vi "EXP 1.vi"() -> ()   [LabVIEW 2018]
panel:
  out "power consumed\n       WATTS":dbl
  out "OVERALL TIIME M.SECS":i32
  out "Alert C2":string
  out "Alert L1":string
  out "Alert L2":string
  out "alertc1":string
  out "Alaramc2":bool
  out "alaraml1":bool
  out "Alaraml2":bool
  out "Alaramc1":bool
  in  "stop 2":bool
  out "LIGHT1 5 POWER":dbl
  out "LIGHT1 4 POWER":dbl
  out "LIGHT23 POWER":dbl
  out "LIGHT1 2 POWER":dbl
  out "OVERALL ENERGY\nCONSUMED":dbl
  out "LAB-1 OVERALL POWER":dbl
  out "LAB-1 OVERALL TIME":i32
  out "LAB-2 OVERALL POWER":dbl
  out "LAB-2 OVERALL TIME":i32
  out "LIGHT 12 TIME":i32 format="%<%H:%M>t"
  out "LIGHT23 TIME":i32 format="%<%H:%M>t"
  out "LIGHT1 4 TIME":i32 format="%<%H:%M>t"
  out "LIGHT1 5 TIME":i32 format="%<%H:%M>t"
  out "FAN13 POWER":dbl
  out "FAN3 POWER":dbl
  out "FAN15 POWER":dbl
  out "FAN5 POWER":dbl
  out "FAN5 TIME":i32
  out "FAN1 5 TIME":i32
  out "FAN3 TIME":i32
  out "FAN13 TIME":i32
  out "FAN1 4":dbl
  out "FAN4":dbl
  out "LIGHT23 2":dbl
  out "LIGHT1 3":dbl
  out "FAN1 4 TIME":i32
  out "FAN4 TIME":i32
  out "LIGHT23 2 TIME":i32
  out "LIGHT 1 3 TIME":i32
  out "CLASS-2 OVERALL TIIME":i32
  out "CLASS-2 POWER OUTPUT":dbl
  out "DAY":string
  out "lighht1 5":bool
  out "lighht1 4":bool
  out "fan 5":bool
  out "fan1 5":bool
  out "light23 2":bool
  out "lighht1 3":bool
  out "fan 4":bool
  out "fan1 4":bool
  out "light23":bool
  out "lighht1 2":bool
  out "fan 3":bool
  out "fan1 3":bool
  out "current time":timestamp
  out "INDICATED VALUE":dbl
  out "light 2 time\nHH:MM 2":i32 caption="light 2 time" format="%<%H:%M>t"
  out "light 1 time\nHH:MM  2":i32 caption="light 2 time" format="%<%H:%M>t"
  out "fan 1 time\nHH:MM   2":i32 caption="light 2 time" format="%<%H:%M>t"
  out "fan 2 time\nHH:MM  2":i32 caption="light 2 time" format="%<%H:%M>t"
  out "light 2 output 2":dbl
  out "light 1 output  2":dbl
  out "fan 1 output  2":dbl
  out "fan 2 output  2":dbl
  out "Alert Overall":string
  out "CLASS 1 OVERALL TIME\nHH:MM  2":i32 caption="light 2 time" format="%<%H:%M>t"
  out "CLASS-1 POWER OUTPUT":dbl
  out "ALARM INDICATOR":bool
  out "light2 2":bool
  out "lighht1":bool
  out "fan 2":bool
  out "fan1 2":bool
  # "PRE"
  # "LAB-1"
  # "CLASS-1 DATA"
  # "CLASS 2"
  # "CLASS1"
  # "LAB-2"
  # "###############################################################"
  # "LAB-1 DATA"
  # "###############################################################"
  # "LAB-2"
  # "#\n#\n#\n#\n#\n#\n#\n#\n#\n#\n#\n#\n#\n#\n#\n#\n#\n#\n#\n#\n#\n#\n#\n#\n#\n#\n#\n#\n#\n#"
  # "##TIME AND POWER OF INDIVIDUAL CLASS ROOMS AND LABS##"
  # "###############################################################"
  # "CLASS-2"
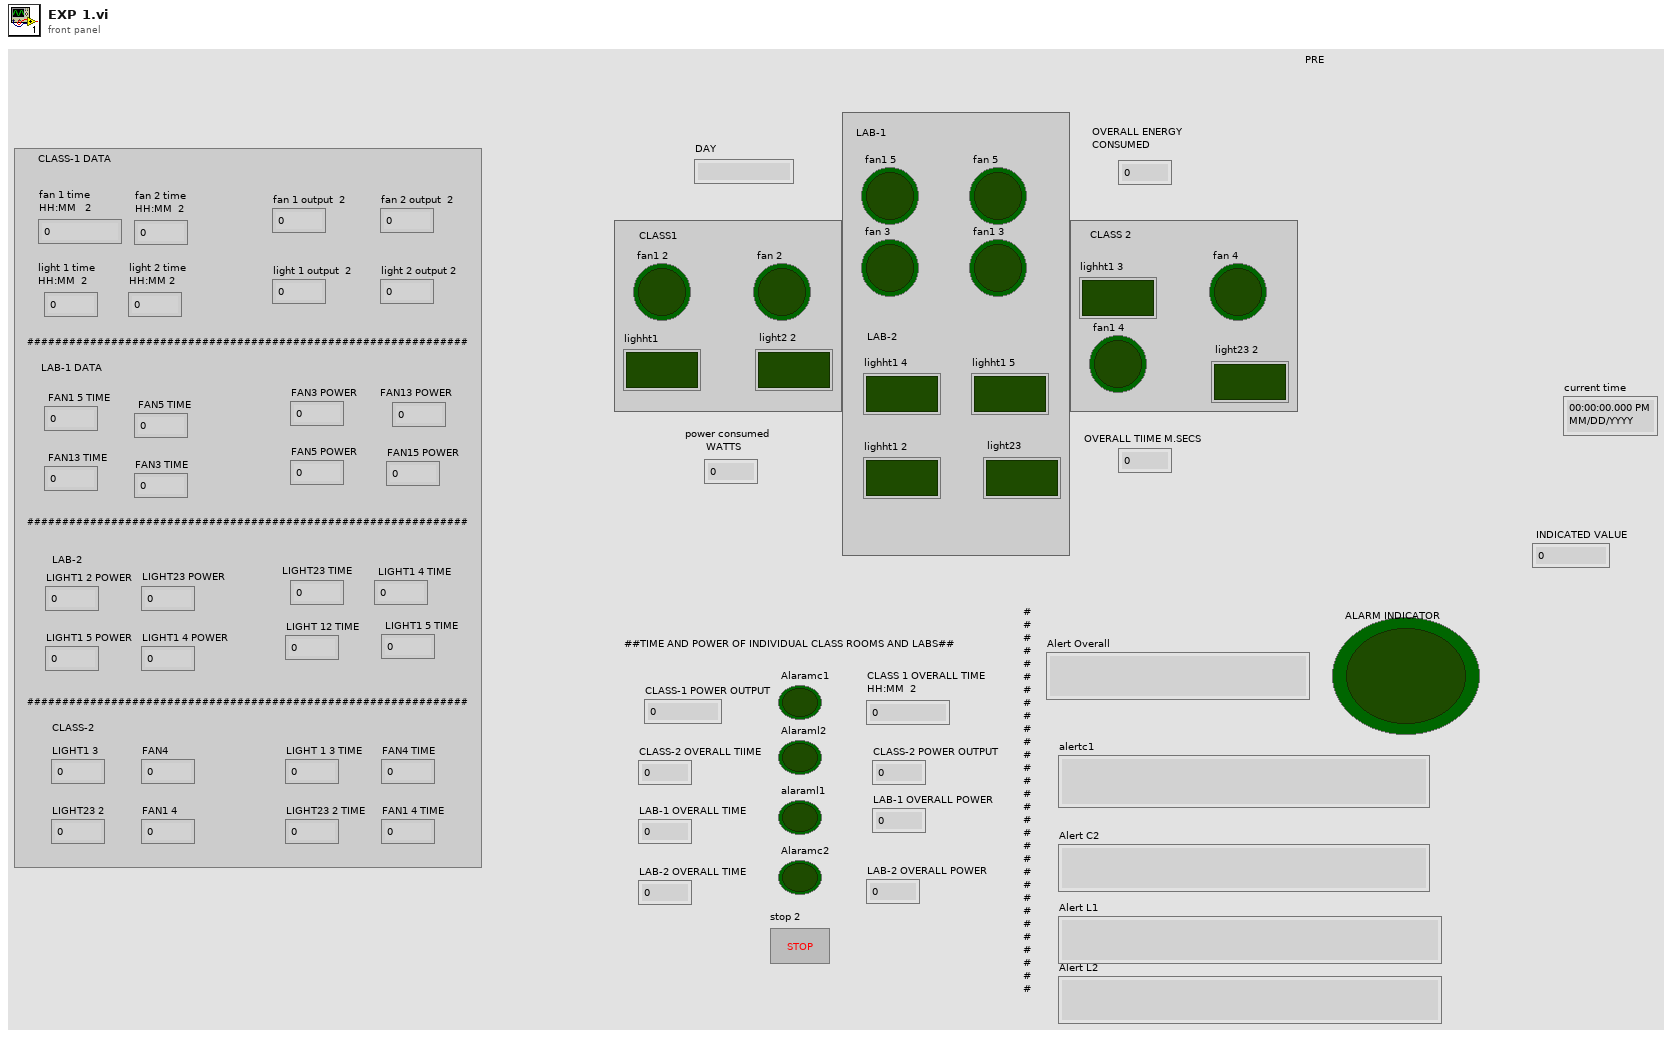
[diagram p1: front panel]
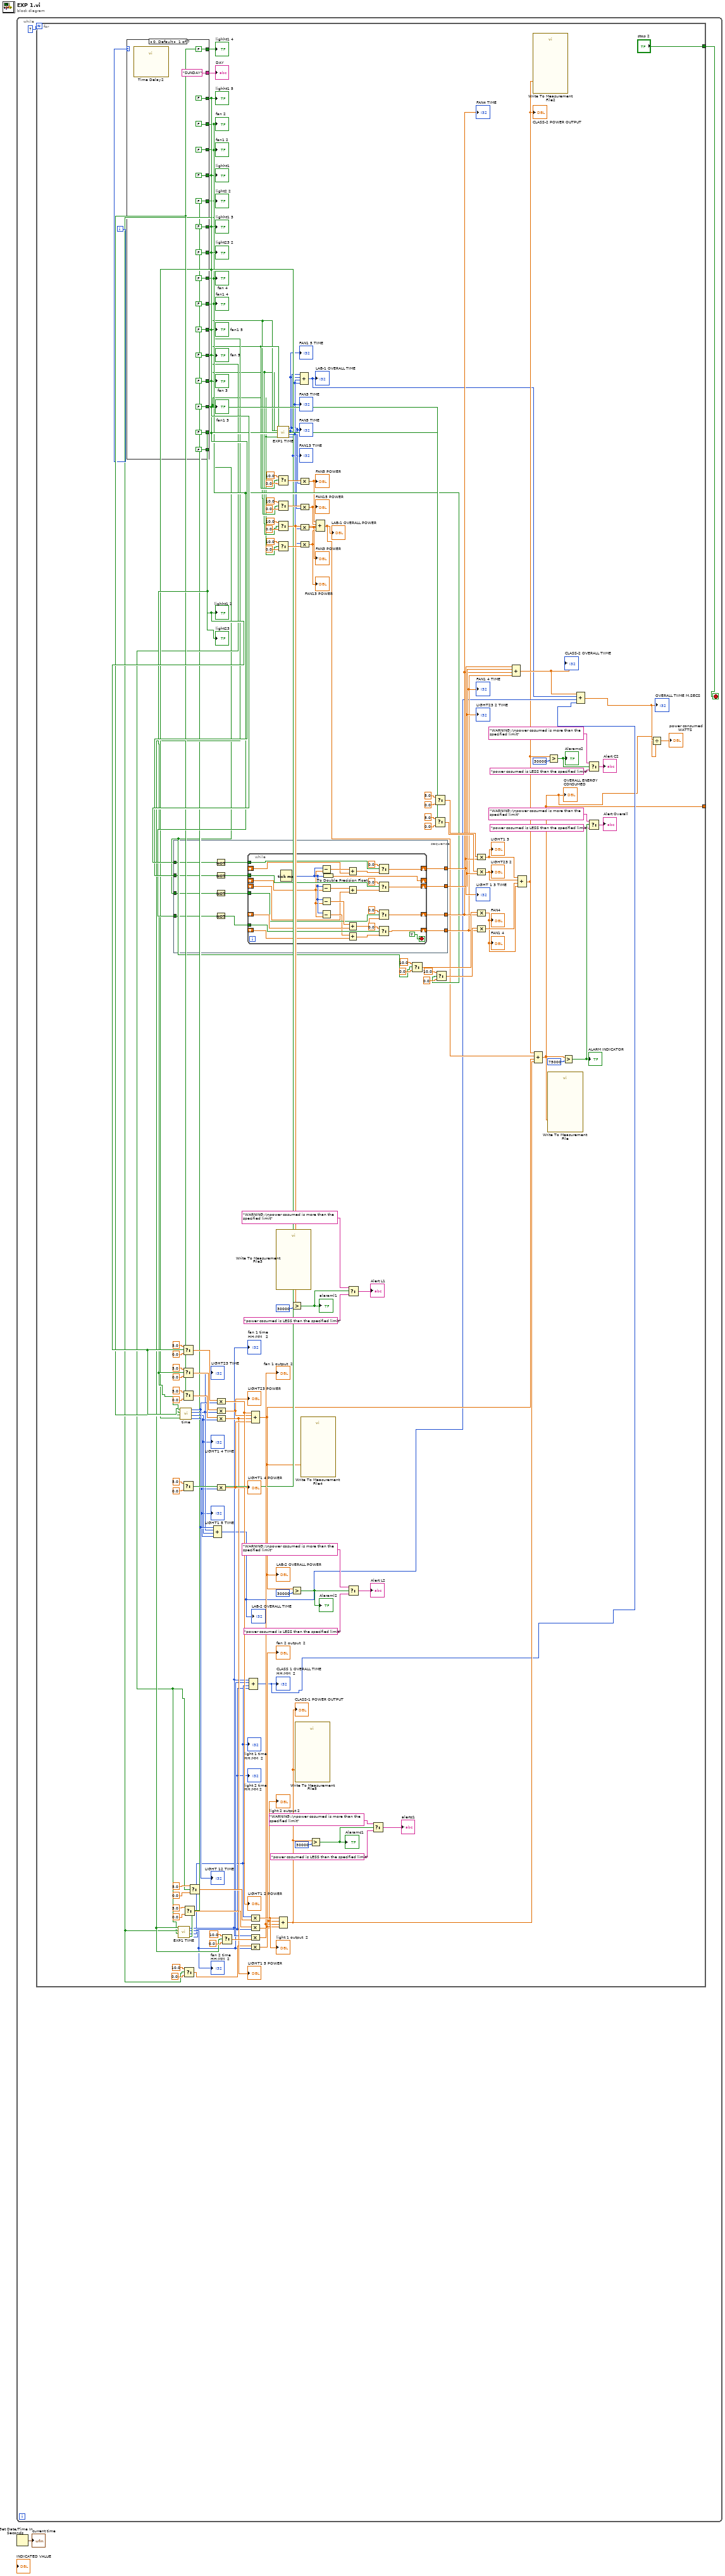
[diagram p0: block diagram]
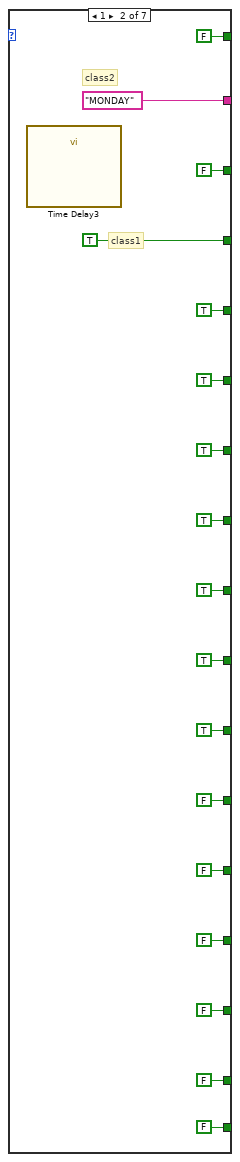
[diagram p2: hidden frame]
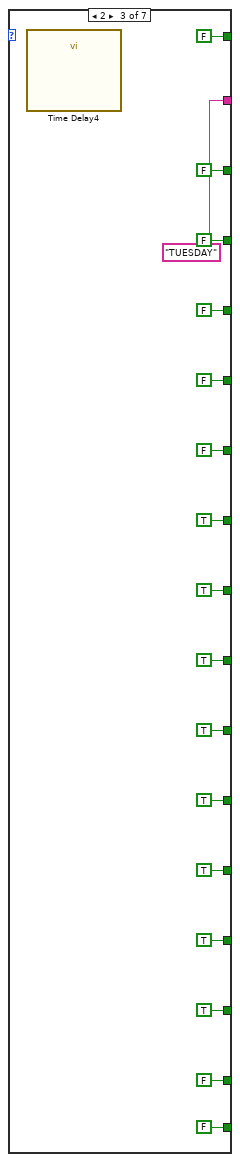
[diagram p3: hidden frame]
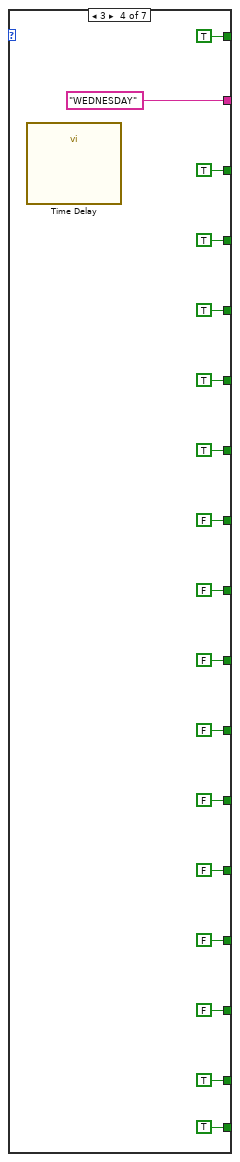
[diagram p4: hidden frame]
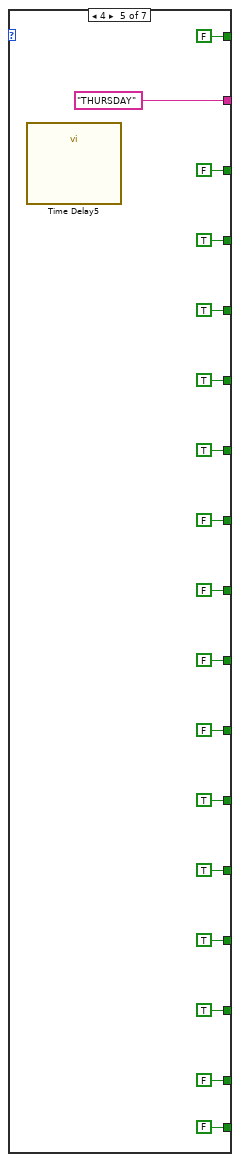
[diagram p5: hidden frame]
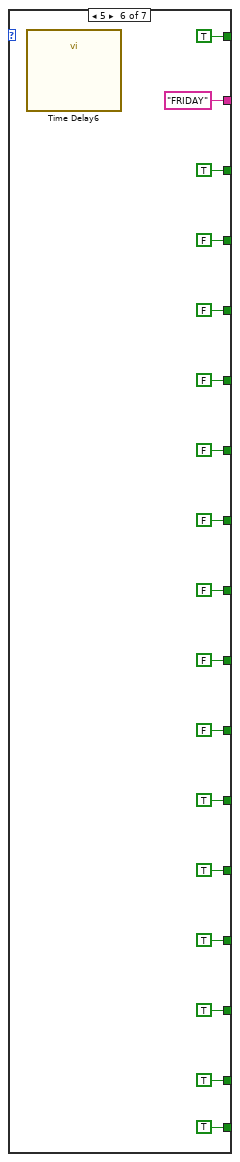
[diagram p6: hidden frame]
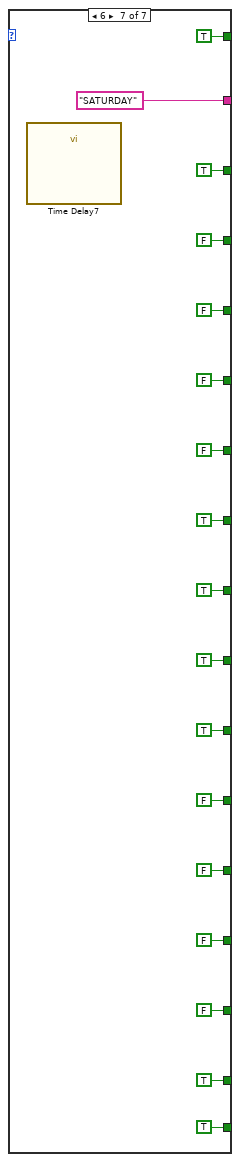
[diagram p7: hidden frame]
diagram:
  n1 = while {
    stop <- w2 stop-if-true
    n2 = for {
      N: 7 -> [_]
      tunnel: [w16] -> _
      tunnel: ["stop 2"] -> w2
      i -> [w54]
      n3 = case shown="0, Default" w54 {
        tunnel: [FALSE ("Boolean 9") TRUE ("Boolean 9") FALSE ("Boolean 9") TRUE ("Boolean 9") TRUE ("Boolean 8") FALSE ("Boolean 8") FALSE ("Boolean 8")] -> w53
        tunnel: [FALSE ("Boolean 11") TRUE ("Boolean 8") FALSE ("Boolean 11") TRUE ("Boolean 11") TRUE ("Boolean 8") FALSE ("Boolean 8") FALSE ("Boolean 8")] -> w52
        tunnel: [FALSE ("Boolean 8") TRUE ("Boolean 11") FALSE ("Boolean 8") TRUE ("Boolean 8") TRUE ("Boolean 8") FALSE ("Boolean 8") FALSE ("Boolean 8")] -> w51
        tunnel: [FALSE ("Boolean 10") TRUE ("Boolean 10") FALSE ("Boolean 10") TRUE ("Boolean 10") TRUE ("Boolean 8") FALSE ("Boolean 8") FALSE ("Boolean 8")] -> w50
        tunnel: [FALSE ("Boolean 8") TRUE ("Boolean 9") TRUE ("Boolean 9") FALSE ("Boolean 8") FALSE ("Boolean 8") FALSE ("Boolean 8") TRUE ("Boolean 8")] -> w110
        tunnel: [FALSE ("Boolean 8") TRUE ("Boolean 9") TRUE ("Boolean 9") FALSE ("Boolean 8") FALSE ("Boolean 8") FALSE ("Boolean 8") TRUE ("Boolean 8")] -> w109
        tunnel: [FALSE ("Boolean 8") TRUE ("Boolean 8") TRUE ("Boolean 8") FALSE ("Boolean 8") FALSE ("Boolean 8") FALSE ("Boolean 8") TRUE ("Boolean 8")] -> w6
        tunnel: [FALSE ("Boolean 8") TRUE ("Boolean 8") TRUE ("Boolean 8") FALSE ("Boolean 8") FALSE ("Boolean 8") FALSE ("Boolean 8") TRUE ("Boolean 8")] -> w88
        tunnel: [FALSE ("Boolean 9") FALSE ("Boolean 9") TRUE ("Boolean 9") FALSE ("Boolean 9") TRUE ("Boolean 8") TRUE ("Boolean 8") FALSE ("Boolean 8")] -> w13
        tunnel: [FALSE ("Boolean 9") FALSE ("Boolean 9") TRUE ("Boolean 9") FALSE ("Boolean 9") TRUE ("Boolean 8") TRUE ("Boolean 8") FALSE ("Boolean 8")] -> w14
        tunnel: [FALSE ("Boolean 9") FALSE ("Boolean 9") TRUE ("Boolean 9") FALSE ("Boolean 9") TRUE ("Boolean 8") TRUE ("Boolean 8") FALSE ("Boolean 8")] -> w12
        tunnel: [FALSE ("Boolean 9") FALSE ("Boolean 9") TRUE ("Boolean 9") FALSE ("Boolean 9") TRUE ("Boolean 8") TRUE ("Boolean 8") FALSE ("Boolean 8")] -> w11
        tunnel: [FALSE ("Boolean 8") FALSE ("Boolean 8") FALSE ("Boolean 8") TRUE ("Boolean 8") FALSE ("Boolean 8") TRUE ("Boolean 8") TRUE ("Boolean 8")] -> w75
        tunnel: [FALSE ("Boolean 8") FALSE ("Boolean 8") FALSE ("Boolean 8") TRUE ("Boolean 8") FALSE ("Boolean 8") TRUE ("Boolean 8") TRUE ("Boolean 8")] -> w74
        tunnel: [FALSE ("Boolean 8") FALSE ("Boolean 8") FALSE ("Boolean 8") TRUE ("Boolean 8") FALSE ("Boolean 8") TRUE ("Boolean 8") TRUE ("Boolean 8")] -> w73
        tunnel: [FALSE ("Boolean 8") FALSE ("Boolean 8") FALSE ("Boolean 8") TRUE ("Boolean 8") FALSE ("Boolean 8") TRUE ("Boolean 8") TRUE ("Boolean 8")] -> w72
        tunnel: ["SUNDAY" "MONDAY" "TUESDAY" "WEDNESDAY" "THURSDAY" "FRIDAY" "SATURDAY"] -> w119
        frame 0, Default {
          n4 = call "Time Delay2"() -> ()  [unwired: 11 in, 1 out]
        }
        frame 1 {
          # "class2"
          # "class1"
          n5 = call "Time Delay3"() -> ()  [unwired: 11 in, 1 out]
        }
        frame 2 {
          n6 = call "Time Delay4"() -> ()  [unwired: 11 in, 1 out]
        }
        frame 3 {
          n7 = call "Time Delay"() -> ()  [unwired: 11 in, 1 out]
        }
        frame 4 {
          n8 = call "Time Delay5"() -> ()  [unwired: 11 in, 1 out]
        }
        frame 5 {
          n9 = call "Time Delay6"() -> ()  [unwired: 11 in, 1 out]
        }
        frame 6 {
          n10 = call "Time Delay7"() -> ()  [unwired: 11 in, 1 out]
        }
      }
      "fan1 2" <- w53
      "fan 2" <- w52
      "lighht1" <- w51
      "light2 2" <- w50
      "fan1 3" <- w11
      "fan 3" <- w12
      "lighht1 2" <- w75
      "light23" <- w74
      "fan1 4" <- w88
      "fan 4" <- w6
      "lighht1 3" <- w110
      "light23 2" <- w109
      "fan1 5" <- w13
      "fan 5" <- w14
      "lighht1 4" <- w73
      "lighht1 5" <- w72
      "DAY" <- w119
      n11 = stacked-sequence {
        tunnel: [w148] -> w97
        tunnel: [w139] -> w98
        tunnel: [w150] -> w99
        tunnel: [w149] -> w100
        tunnel: w88 -> [w142]
        tunnel: w6 -> [w140]
        tunnel: w109 -> [w144]
        tunnel: w110 -> [w143]
        frame #0 {
          n12 = Not(x=w143) -> (.not. x?=w146:bool)
          n13 = Not(x=w144) -> (.not. x?=w147:bool)
          n14 = Not(x=w140) -> (.not. x?=w141:bool)
          n15 = Not(x=w142) -> (.not. x?=w145:bool)
          n16 = while {
            shift-right: [w165] -> w139
            shift-left: _ -> [w177]
            shift-right: [w175] -> _
            shift-left: _ -> [w151]
            tunnel: w141 -> [w173]
            tunnel: w145 -> [w169]
            tunnel: w146 -> [w168]
            tunnel: w147 -> [w167]
            shift-right: [w164] -> w148
            shift-left: _ -> [w158]
            shift-right: [w163] -> w149
            shift-left: _ -> [w156]
            shift-right: [w162] -> w150
            shift-left: _ -> [w154]
            stop <- TRUE stop-if-true
            n17 = Tick Count (ms)() -> (millisecond timer value=w152:u32)
            n18 = Subtract(x=w152, y=w151) -> (x-y=w161:dbl)
            n19 = Subtract(x=w152, y=w151) -> (x-y=w160:dbl)
            n20 = Subtract(x=w152, y=w151) -> (x-y=w178:dbl)
            n21 = Subtract(x=w152, y=w151) -> (x-y=w159:dbl)
            n22 = To Double Precision Float(number=w152) -> (double precision float=w175:dbl)
            n23 = Add(x=w161, y=w156) -> (x+y=w155:dbl)
            n24 = Add(x=w160, y=w154) -> (x+y=w153:dbl)
            n25 = Add(x=w178, y=w177) -> (x+y=w166:dbl)
            n26 = Add(x=w159, y=w158) -> (x+y=w157:dbl)
            n27 = Select(t=0.0, s=w168, f=w155) -> (s? t:f=w163:dbl)
            n28 = Select(t=0.0, s=w167, f=w153) -> (s? t:f=w162:dbl)
            n29 = Select(t=0.0, s=w173, f=w166) -> (s? t:f=w165:dbl)
            n30 = Select(t=0.0, s=w169, f=w157) -> (s? t:f=w164:dbl)
          }
        }
      }
      "LIGHT 1 3 TIME" <- w100
      "LIGHT23 2 TIME" <- w99
      "FAN4 TIME" <- w98
      "FAN1 4 TIME" <- w97
      n31 = call "EXP1 TIME.vi"("s 2"=w50, "s"=w51, "s 4"=w52, "s 3"=w53) -> ("time 2"=w46:i32, "time"=w47:i32, "time 4"=w48:i32, "time 3"=w49:i32)  [unwired: 4 in]
      "fan 1 time\nHH:MM   2" <- w49
      "fan 2 time\nHH:MM  2" <- w48
      "light 1 time\nHH:MM  2" <- w47
      "light 2 time\nHH:MM 2" <- w46
      n32 = call "time.vi"("s 2"=w72, "s"=w73, "s 4"=w74, "s 3"=w75) -> ("time 2"=w61:i32, "time"=w62:i32, "time 4"=w63:i32, "time 3"=w64:i32)  [unwired: 4 in]
      "LIGHT1 5 TIME" <- w61
      "LIGHT1 4 TIME" <- w62
      "LIGHT23 TIME" <- w63
      "LIGHT 12 TIME" <- w64
      n33 = Select(t=5.0, s=w75, f=0.0) -> (s? t:f=w71:dbl)
      n34 = Select(t=5.0, s=w74, f=0.0) -> (s? t:f=w70:dbl)
      n35 = Select(t=5.0, s=w73, f=0.0) -> (s? t:f=w69:dbl)
      n36 = Select(t=5.0, s=w72, f=0.0) -> (s? t:f=w68:dbl)
      n37 = Select(t=10.0, s=w52, f=0.0) -> (s? t:f=w55:dbl)
      n38 = Select(t=5.0, s=w50, f=0.0) -> (s? t:f=w56:dbl)
      n39 = Select(t=5.0, s=w51, f=0.0) -> (s? t:f=w136:dbl)
      n40 = Compound Arithmetic op=ADD(w64, w63, w62, w61) -> (w20:i32)
      "LAB-2 OVERALL TIME" <- w20
      n41 = Compound Arithmetic op=MULTIPLY(w71, w64) -> (w60:dbl)
      "LIGHT1 2 POWER" <- w60
      n42 = Compound Arithmetic op=MULTIPLY(w70, w63) -> (w59:dbl)
      "LIGHT23 POWER" <- w59
      n43 = Compound Arithmetic op=MULTIPLY(w69, w62) -> (w57:dbl)
      "LIGHT1 5 POWER" <- w57
      n44 = Compound Arithmetic op=MULTIPLY(w68, w61) -> (w58:dbl)
      "LIGHT1 4 POWER" <- w58
      n45 = Select(t=10.0, s=w53, f=0.0 ("t")) -> (s? t:f=w132:dbl)
      n46 = Compound Arithmetic op=ADD(w49, w48, w47, w46) -> (w19:i32)
      "CLASS 1 OVERALL TIME\nHH:MM  2" <- w19
      n47 = Compound Arithmetic op=ADD(w60, w59, w57, w58) -> (w23:dbl)
      "LAB-2 OVERALL POWER" <- w23
      n48 = Compound Arithmetic op=MULTIPLY(w47, w136) -> (w137:dbl)
      "light 1 output  2" <- w137
      n49 = Compound Arithmetic op=MULTIPLY(w56, w46) -> (w133:dbl)
      "light 2 output 2" <- w133
      n50 = Compound Arithmetic op=MULTIPLY(w49, w132) -> (w134:dbl)
      "fan 1 output  2" <- w134
      n51 = Compound Arithmetic op=MULTIPLY(w55, w48) -> (w135:dbl)
      "fan 2 output  2" <- w135
      n52 = call "EXP1 TIME.vi"("s 2"=w11, "s"=w12, "s 4"=w13, "s 3"=w14) -> ("time 2"=w8:i32, "time"=w9:i32, "time 4"=w5:i32, "time 3"=w10:i32)  [unwired: 4 in]
      "FAN13 TIME" <- w8
      "FAN3 TIME" <- w9
      "FAN1 5 TIME" <- w5
      "FAN5 TIME" <- w10
      n53 = Select(t=10.0, s=w14, f=0.0) -> (s? t:f=w79:dbl)
      n54 = Select(t=10.0, s=w13, f=0.0) -> (s? t:f=w78:dbl)
      n55 = Select(t=10.0, s=w12, f=0.0) -> (s? t:f=w77:dbl)
      n56 = Select(t=10.0, s=w11, f=0.0) -> (s? t:f=w76:dbl)
      n57 = Compound Arithmetic op=ADD(w137, w133, w134, w135) -> (w22:dbl)
      "CLASS-1 POWER OUTPUT" <- w22
      n58 = Greater?(x=w23, y=30000) -> (0:w35:bool)
      "Alaraml2" <- w35
      n59 = call "Write To Measurement File5"("Signals"=w22) -> ()  [unwired: 16 in, 3 out]
      n60 = Compound Arithmetic op=ADD(w10, w5, w9, w9) -> (w7:i32)
      "LAB-1 OVERALL TIME" <- w7
      n61 = Compound Arithmetic op=MULTIPLY(w79, w10) -> (w67:dbl)
      "FAN5 POWER" <- w67
      n62 = Compound Arithmetic op=MULTIPLY(w78, w5) -> (w66:dbl)
      "FAN15 POWER" <- w66
      n63 = Compound Arithmetic op=MULTIPLY(w77, w9) -> (w65:dbl)
      "FAN3 POWER" <- w65
      n64 = Compound Arithmetic op=MULTIPLY(w8, w76) -> (w4:dbl)
      "FAN13 POWER" <- w4
      n65 = call "Write To Measurement File4"("Signals"=w23) -> ()  [unwired: 16 in, 3 out]
      n66 = Greater?(x=w22, y=30000) -> (0:w40:bool)
      "Alaramc1" <- w40
      n67 = Compound Arithmetic op=ADD(w67, w66, w65, w4) -> (w24:dbl)
      "LAB-1 OVERALL POWER" <- w24
      n68 = call "Write To Measurement File3"("Signals"=w24) -> ()  [unwired: 16 in, 3 out]
      n69 = Greater?(x=w24, y=30000) -> (0:w30:bool)
      "alaraml1" <- w30
      n70 = Select(t="WARNING::\npower cosumed is more than the specified limit", s=w30, f="power cosumed is LESS than the specified limit") -> (s? t:f=→"Alert L1":string)
      n71 = Select(t="WARNING::\npower cosumed is more than the specified limit", s=w35, f="power cosumed is LESS than the specified limit") -> (s? t:f=→"Alert L2":string)
      n72 = Select(t="WARNING::\npower cosumed is more than the specified limit", s=w40, f="power cosumed is LESS than the specified limit") -> (s? t:f=→"alertc1":string)
      n73 = Select(t=10.0, s=w6, f=0.0) -> (s? t:f=w106:dbl)
      n74 = Select(t=5.0, s=w109, f=0.0) -> (s? t:f=w108:dbl)
      n75 = Select(t=5.0, s=w110, f=0.0) -> (s? t:f=w107:dbl)
      n76 = Select(t=10.0, s=w88, f=0.0) -> (s? t:f=w105:dbl)
      n77 = Compound Arithmetic op=MULTIPLY(w108, w100) -> (w104:dbl)
      "LIGHT1 3" <- w104
      n78 = Compound Arithmetic op=MULTIPLY(w107, w99) -> (w103:dbl)
      "LIGHT23 2" <- w103
      n79 = Compound Arithmetic op=MULTIPLY(w106, w98) -> (w102:dbl)
      "FAN4" <- w102
      n80 = Compound Arithmetic op=MULTIPLY(w105, w97) -> (w101:dbl)
      "FAN1 4" <- w101
      n81 = Compound Arithmetic op=ADD(w100, w99, w98, w97) -> (w21:dbl)
      "CLASS-2 OVERALL TIIME" <- w21
      n82 = Compound Arithmetic op=ADD(w104, w103, w102, w101) -> (w18:dbl)
      "CLASS-2 POWER OUTPUT" <- w18
      n83 = call "Write To Measurement File2"("Signals"=w18) -> ()  [unwired: 16 in, 3 out]
      n84 = Compound Arithmetic op=ADD(w18, w24, w23, w22) -> (w16:dbl)
      "OVERALL ENERGY\nCONSUMED" <- w16
      n85 = call "Write To Measurement File"("Signals"=w16) -> ()  [unwired: 16 in, 3 out]
      n86 = Greater?(x=w18, y=30000) -> (0:w25:bool)
      "Alaramc2" <- w25
      n87 = Greater?(x=w16, y=75000) -> (0:w131:bool)
      "ALARM INDICATOR" <- w131
      n88 = Compound Arithmetic op=ADD(w21, w7, w20, w19) -> (w15:dbl)
      "OVERALL TIIME M.SECS" <- w15
      n89 = Select(t="WARNING::\npower cosumed is more than the specified limit", s=w25, f="power cosumed is LESS than the specified limit") -> (s? t:f=→"Alert C2":string)
      n90 = Select(t="WARNING::\npower cosumed is more than the specified limit", s=w131, f="power cosumed is LESS than the specified limit") -> (s? t:f=→"Alert Overall":string)
      n91 = Divide(x=w16, y=w15) -> (x/y=→"power consumed\n       WATTS":dbl)
    }
  }
  n92 = Get Date/Time In Seconds() -> (seconds since 1Jan1904=→"current time":timestamp)
